vi "plot focus curve.vi"(8 "error in (no error)":errorcluster, 11 "Autofocus in":refnum<class "Autofocus.lvclass">) -> (0 "error out":errorcluster, 1 "x array":dbl[](array[numeric]), 2 "y array":dbl[](array[numeric]), 3 "Autofocus out":refnum<class "Autofocus.lvclass">)   [LabVIEW 2012, in "Autofocus.lvclass"]
uses:
  Autofocus.lvclass
  Autofocus.lvclass/Autofocus.ctl
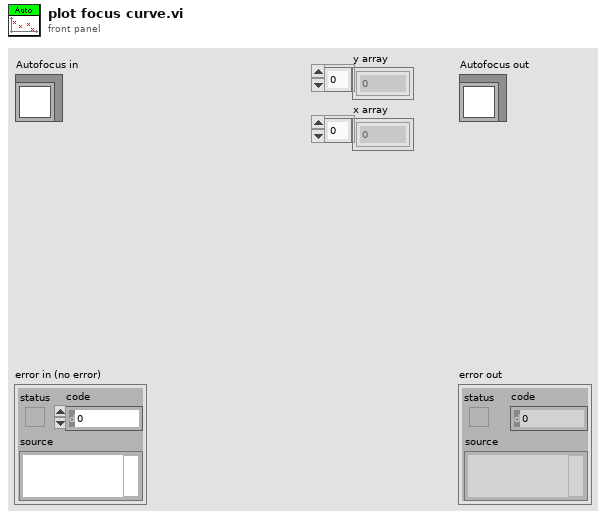
[diagram p1: front panel]
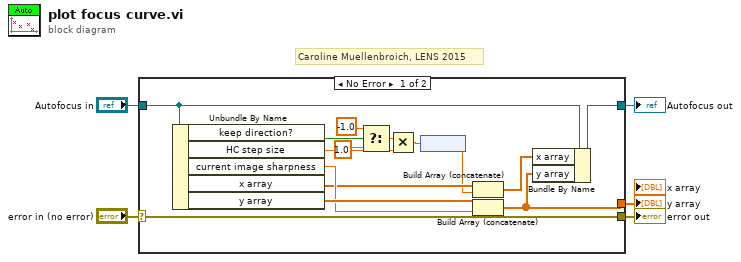
[diagram p0: block diagram]
diagram:
  # "Caroline Muellenbroich, LENS 2015"
  n1 = case shown="No Error" "error in (no error)" {
    selector: "error in (no error)" -> [w20 w22]
    tunnel: [w20 w22] -> w4
    tunnel: [w13 w21] -> w2
    tunnel: "Autofocus in" -> [w14 w21]
    tunnel: [w9 _] -> w1
    frame No Error {
      n2 = Unbundle By Name(w14) -> ("keep direction?"=w17:bool, "HC step size"=w15:dbl[unit], "current image sharpness"=w10:dbl, "x array"=w7:dbl[], "y array"=w11:dbl[])
      n3 = Select(t=-1.0 ("y"), s=w17, f=1.0 ("y")) -> (s? t:f=w16:dbl)
      n4 = Multiply(x=w16, y=w15) -> (x*y=w12:dbl[unit])
      n5 = node(w12) -> (w6:dbl)
      n6 = Build Array (concatenate)(w7, w6) -> (w8:dbl[])
      n7 = Build Array (concatenate)(w11, w10) -> (w9:dbl[])
      n8 = Bundle By Name(cluster=w14, "x array"=w8, "y array"=w9) -> (w13:refnum<class "Autofocus.lvclass">)
    }
    frame Error {
    }
  }
  "error out" <- w4
  "Autofocus out" <- w2
  "y array" <- w1
